vi "CleanUp.vi"(8 "Error In":errorcluster, 11 "WebView in":refnum<class "WebView.lvclass">) -> (0 "Error Out":errorcluster)   [LabVIEW 2024, in "WebView.lvclass"]
uses:
  WebView.lvclass
  WebView.lvclass/WebView.ctl
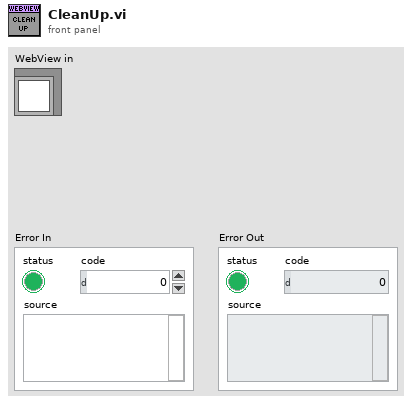
[diagram p1: front panel]
types:
  T1 = typedef "WebView.lvclass/Events--cluster.ctl" = cluster{"Navigation Complete Event":refnum<user-event>, "Source Changed Event":refnum<user-event>, "Document Title Changed Event":refnum<user-event>, "Status Bar Text Changed":refnum<user-event>, "Web Message Received":refnum<user-event>, "Window Close Requested":refnum<user-event>, "DOM Loaded":refnum<user-event>, "Navigation Started Event":refnum<user-event>}
  T2 = typedef "WebView.lvclass/Resources--cluster.ctl" = cluster{"WebView2 Control":refnum<k24>, "Webview2 Core":refnum<k24>, "event callback":refnum<k27>, "Environment":refnum<k24>}
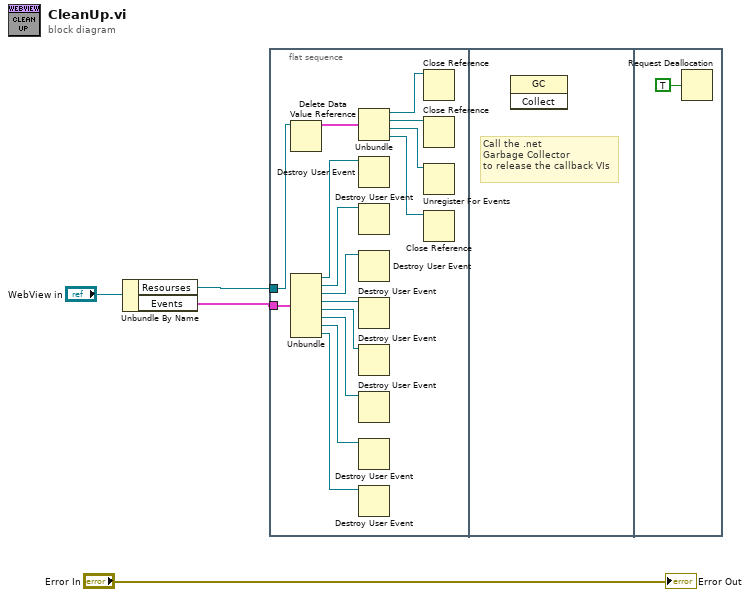
[diagram p0: block diagram]
diagram:
  n1 = Unbundle By Name("WebView in") -> ("Resourses"=w3:refnum<data-value>, "Events"=w2:T1)
  n2 = flat-sequence {
    tunnel: w3 -> [w8]
    tunnel: w2 -> [w19]
    frame #0 {
      n3 = Delete Data Value Reference(data value reference=w8) -> (data value=w7:T2)  [unwired: 1 in, 1 out]
      n4 = Unbundle(w19) -> ("Navigation Complete Event"=w18:refnum<user-event>, "Source Changed Event"=w17:refnum<user-event>, "Document Title Changed Event"=w16:refnum<user-event>, "Status Bar Text Changed"=w15:refnum<user-event>, "Web Message Received"=w14:refnum<user-event>, "Window Close Requested"=w13:refnum<user-event>, "DOM Loaded"=w12:refnum<user-event>, "Navigation Started Event"=w11:refnum<user-event>)
      n5 = Unbundle(w7) -> ("WebView2 Control"=w10:refnum<k24>, "Webview2 Core"=w9:refnum<k24>, "event callback"=w6:refnum<k27>, "Environment"=w5:refnum<k24>)
      n6 = Destroy User Event(user event=w18) -> ()  [unwired: 1 in, 1 out]
      n7 = Destroy User Event(user event=w17) -> ()  [unwired: 1 in, 1 out]
      n8 = Destroy User Event(user event=w16) -> ()  [unwired: 1 in, 1 out]
      n9 = Destroy User Event(user event=w15) -> ()  [unwired: 1 in, 1 out]
      n10 = Destroy User Event(user event=w14) -> ()  [unwired: 1 in, 1 out]
      n11 = Destroy User Event(user event=w13) -> ()  [unwired: 1 in, 1 out]
      n12 = Destroy User Event(user event=w12) -> ()  [unwired: 1 in, 1 out]
      n13 = Destroy User Event(user event=w11) -> ()  [unwired: 1 in, 1 out]
      n14 = Close Reference(reference=w10) -> ()  [unwired: 1 in, 1 out]
      n15 = Close Reference(reference=w9) -> ()  [unwired: 1 in, 1 out]
      n16 = Unregister For Events(event registration refnum=w6) -> ()  [unwired: 1 in, 1 out]
      n17 = Close Reference(reference=w5) -> ()  [unwired: 1 in, 1 out]
    }
    frame #1 {
      # "Call the .net \nGarbage Collector\nto release the callback VIs"
      n18 = invoke class="GC" method="Collect"() -> ()  [unwired: 3 in, 3 out]
    }
    frame #2 {
      n19 = Request Deallocation(TRUE ("flag")) -> ()
    }
  }
  "Error Out" <- "Error In"
